vi "displayScriptEvents.vi"(8 "error in (no error)":errorcluster, 11 "ActionEditor in":refnum<class "ActionEditor.lvclass">) -> (0 "error out":errorcluster, 3 "ActionEditor out":refnum<class "ActionEditor.lvclass">)   [LabVIEW 2011, in "Views.lvlib" / "ScriptEditor.lvlib" / "ActionEditor.lvclass"]
uses:
  ActionEditor.lvclass
  ActionEditor.lvclass/ActionEditor.ctl
  Tools/Scripting/ScriptingEvent/ScriptEventList/ScriptEventList.lvclass
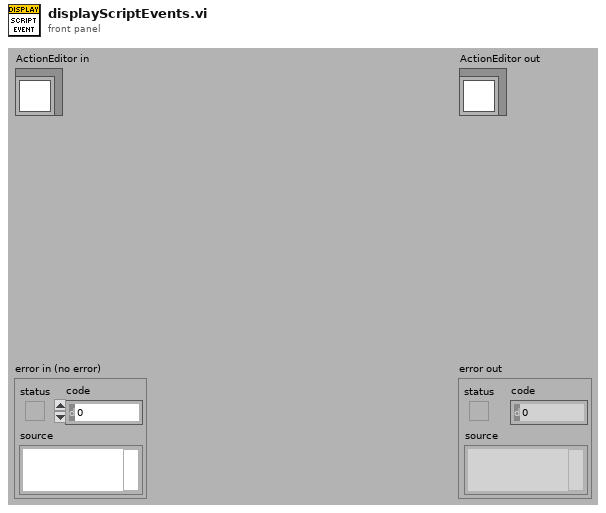
[diagram p1: front panel]
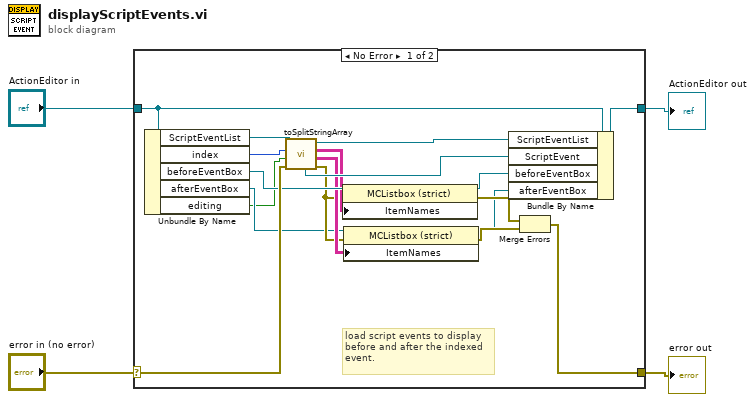
[diagram p0: block diagram]
diagram:
  n1 = case shown="No Error" "error in (no error)" {
    selector: "error in (no error)" -> [w20 w24]
    tunnel: [w6 w24] -> w3
    tunnel: [w18 w23] -> w1
    tunnel: "ActionEditor in" -> [w19 w23]
    frame No Error {
      # "load script events to display\nbefore and after the indexed\nevent."
      n2 = Unbundle By Name(w19) -> ("ScriptEventList"=w22:refnum<class "ScriptEventList.lvclass">, "index"=w21:i32, "beforeEventBox"=w15:refnum<vi>, "afterEventBox"=w10:refnum<vi>, "editing"=w5:bool)
      n3 = call "toSplitStringArray.vi"("error in (no error)"=w20, "editing?"=w5, "splitIndex"=w21, "ScriptEventList in"=w22) -> ("error out"=w11:errorcluster, "AfterIndex"=w12:string[][], "BeforeIndex"=w13:string[][], "ScriptEventList out"=w17:refnum<class "ScriptEventList.lvclass">, "indexedScriptEvent"=w16:refnum<class "ScriptEvent.lvclass">)  [unwired: 3 in]
      n4 = property class="MCListbox (strict)"(reference=w15, error in=w11, "ItemNames"=w13) -> (reference out=w14:refnum<vi>, error out=w9:errorcluster)
      n5 = property class="MCListbox (strict)"(reference=w10, error in=w11, "ItemNames"=w12) -> (reference out=w7:refnum<vi>, error out=w8:errorcluster)
      n6 = Bundle By Name(cluster=w19, "ScriptEventList"=w17, "ScriptEvent"=w16, "beforeEventBox"=w14, "afterEventBox"=w7) -> (w18:refnum<class "ActionEditor.lvclass">)
      n7 = Merge Errors(w9, w8) -> (w6:errorcluster)
    }
    frame Error {
    }
  }
  "error out" <- w3
  "ActionEditor out" <- w1
